vi "Recieving_end_DAQ_data.vi"() -> ()   [LabVIEW 2017]
uses:
  <vilib>/Waveform/DWDTOps.llb/DWDT Binary U16 to Digital.vi
  <vilib>/Waveform/WDTOps.llb/WDT Append Waveforms DBL.vi
panel:
  out "Waveform Chart":waveform(dbl)(graph)
  out "0, 1":i16[](array[numeric])
  out "Boolean array":bool[](array[boolean])
  in  "stop":bool
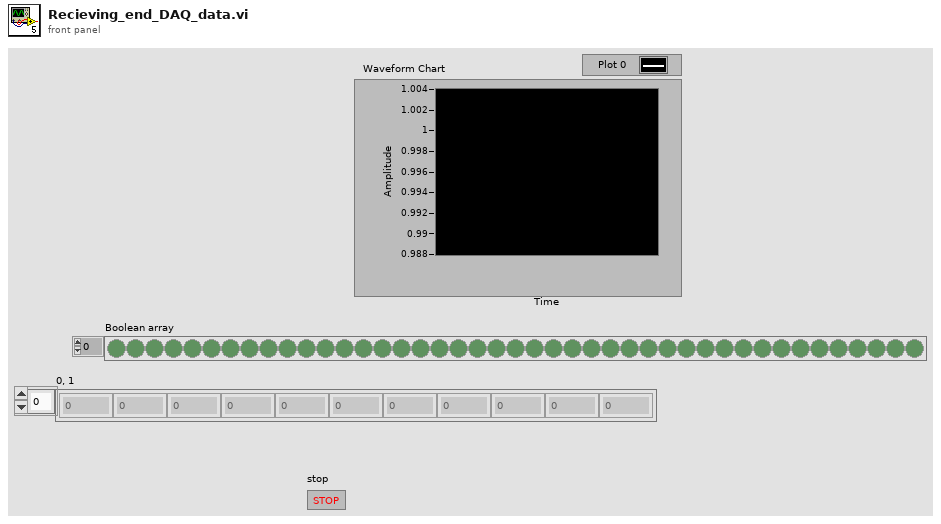
[diagram p1: front panel]
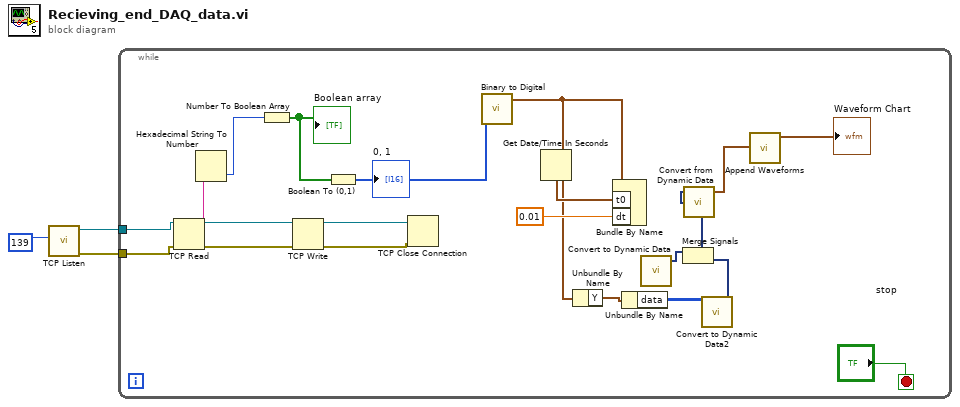
[diagram p0: block diagram]
diagram:
  n1 = call <vilib>:"TCP Listen.vi"("port"=139) -> ("error out"=w2:errorcluster, "connection ID"=w3:refnum<k5>)  [unwired: 6 in, 3 out]
  n2 = while {
    tunnel: w3 -> [w24]
    tunnel: w2 -> [w23]
    stop <- "stop" stop-if-true
    n3 = TCP Read(connection ID=w24, error in (no error)=w23) -> (connection ID out=w22:refnum<k5>, data out=w15:string, error out=w20:errorcluster)  [unwired: 3 in]
    n4 = Hexadecimal String To Number(string=w15) -> (number=w17:u32)  [unwired: 2 in, 1 out]
    n5 = Number To Boolean Array(number=w17) -> (Boolean array=w16:bool[])
    "Boolean array" <- w16
    n6 = TCP Write(connection ID=w22, error in (no error)=w20) -> (connection ID out=w21:refnum<k5>, error out=w19:errorcluster)  [unwired: 2 in, 1 out]
    n7 = Boolean To (0,1)(Boolean=w16) -> (0, 1=w14:i16[])
    "0, 1" <- w14
    n8 = TCP Close Connection(connection ID=w21, error in (no error)=w19) -> ()  [unwired: 1 in, 2 out]
    n9 = call-poly <vilib>:"Binary to Digital.vi"("binary array"=w14) -> ("digital waveform"=w8:digitalwaveform)  [unwired: 9 in, 1 out]
    n10 = Get Date/Time In Seconds() -> (seconds since 1Jan1904=w12:timestamp)
    n11 = Unbundle By Name(w8) -> ("Y"=w7:digitaldata)
    n12 = Bundle By Name(cluster=w8, "t0"=w12, "dt"=0.01) -> ()  [unwired: 1 out]
    n13 = Unbundle By Name(w7) -> ("data"=w5:u8[][])
    n14 = call "Convert to Dynamic Data"() -> ("Dynamic Data Type"=w10:dynamicdata)  [unwired: 4 in]
    n15 = call "Convert to Dynamic Data2"("2D Array"=w5) -> ("Dynamic Data Type"=w4:dynamicdata)  [unwired: 3 in]
    n16 = Merge Signals(w10, w4) -> (w6:dynamicdata)
    n17 = call "Convert from Dynamic Data"("Dynamic Data Type"=w6) -> ("Waveform"=w9:waveform(dbl))  [unwired: 3 in]
    n18 = call-poly <vilib>:"Append Waveforms.vi"("waveform B"=w9) -> ("waveform out"=→"Waveform Chart":waveform(dbl))  [unwired: 9 in, 1 out]
  }
